vi "RGB to LAB.vi"(3 "Blue":dbl, 4 "Green":dbl, 5 "Red":dbl) -> (0 "B":dbl, 1 "A":dbl, 2 "L":dbl)   [LabVIEW 2012]
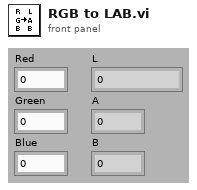
[diagram p1: front panel]
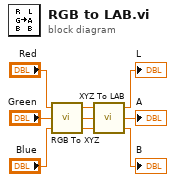
[diagram p0: block diagram]
diagram:
  n1 = call "RGB To XYZ.vi"("Blue"="Blue", "Green"="Green", "Red"="Red") -> ("Z"=w7:dbl, "Y"=w8:dbl, "X"=w9:dbl)
  n2 = call "XYZ To LAB.vi"("Z"=w7, "Y"=w8, "X"=w9) -> ("B"=→"B":dbl, "A"=→"A":dbl, "L"=→"L":dbl)
